vi "GetString.vi"(8 "error in (no error)":errorcluster, 11 "FolloWin in":refnum<class "FolloWin.lvclass">) -> (0 "error out":errorcluster, 2 "String Text":string, 3 "FolloWin out":refnum<class "FolloWin.lvclass">)   [LabVIEW 2023, in "FolloWin.lvclass"]
doc: "Gets the text shown by FolloWin"
uses:
  FolloWin.lvclass
  FolloWin.lvclass/FolloWin.ctl
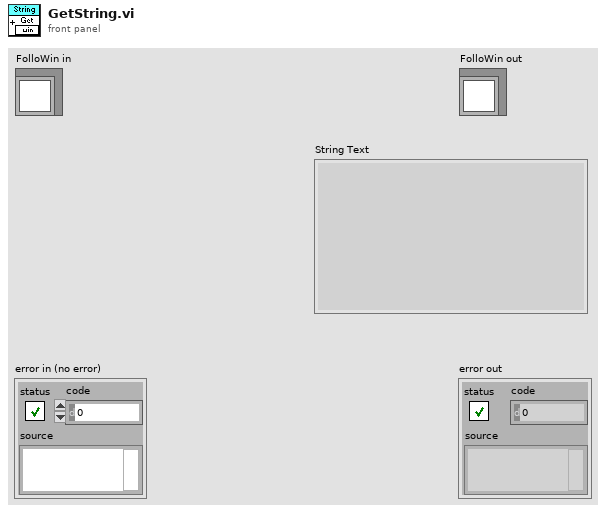
[diagram p1: front panel]
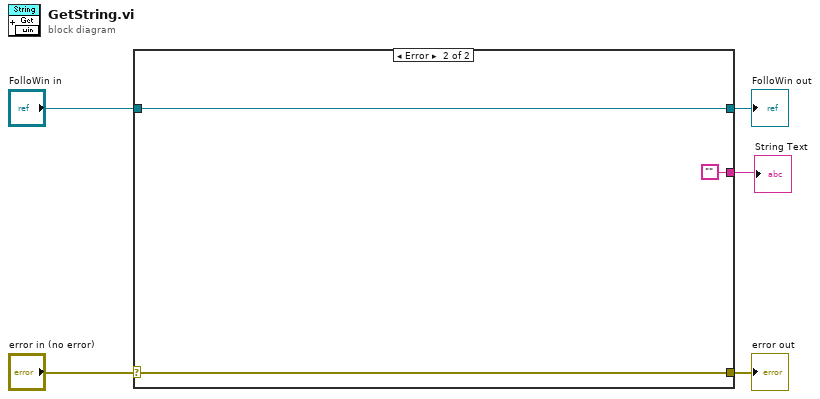
[diagram p0: block diagram]
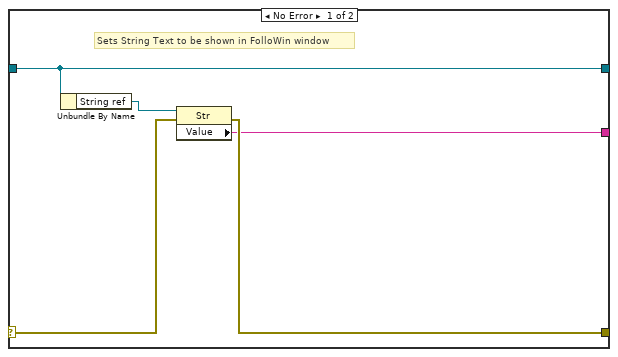
[diagram p2: hidden frame]
diagram:
  n1 = case shown="Error" "error in (no error)" {
    selector: "error in (no error)" -> [w8 w13]
    tunnel: [w7 w13] -> w4
    tunnel: [w10 w12] -> w2
    tunnel: "FolloWin in" -> [w10 w12]
    tunnel: [w6 "" ("Value")] -> w1
    frame No Error {
      # "Sets String Text to be shown in FolloWin window"
      n2 = Unbundle By Name(w10) -> ("String ref"=w9:refnum<vi>)
      n3 = property on="Property Node" class="Str"(reference=w9, error in=w8) -> (error out=w7:errorcluster, "Value"=w6:string)  [unwired: 1 out]
    }
    frame Error {
    }
  }
  "error out" <- w4
  "FolloWin out" <- w2
  "String Text" <- w1
